vi "Unregister Object.vi"(6 "timeout (100 ms)":i32, 11 "Fully Qualified Name":string) -> (0 "timed out":bool)   [LabVIEW 2014, in "UniqueName.lvlib" / "UniqueName.lvclass"]
uses:
  UniqueName.lvclass
  Command.ctl
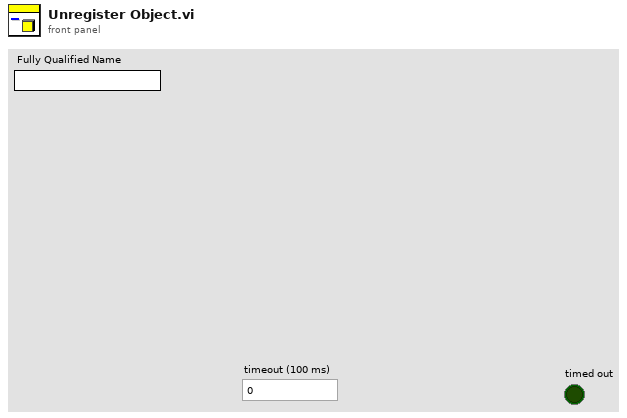
[diagram p1: front panel]
types:
  T1 = typedef "UniqueName.lvlib/UniqueName.lvclass/Command.ctl" = enum16{"Get", "Get All", "Set", "Delete", "Get Status", "Init", "Reserve Ownership", "Release Ownership", "Lock", "Unlock"}
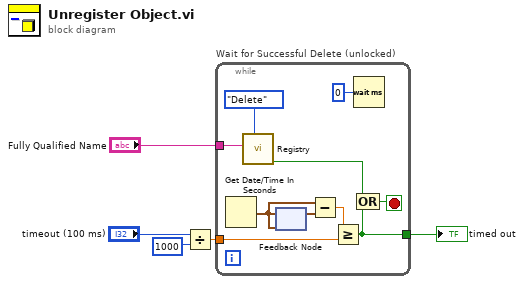
[diagram p0: block diagram]
diagram:
  n1 = Divide(x="timeout (100 ms)", y=1000) -> (x/y=w3:dbl)
  n2 = while "Wait for Successful Delete (unlocked)" {
    tunnel: w3 -> [w13]
    tunnel: [w7] -> w2
    tunnel: "Fully Qualified Name" -> [w6]
    stop <- w14 stop-if-true
    n3 = Get Date/Time In Seconds() -> (seconds since 1Jan1904=w11:timestamp)
    n4 = call "Registry.vi"("Command (Get)"=Command."Delete", "Search term (Get & Delete Operations)"=w6) -> ("Found or Completed?"=w8:bool)  [unwired: 5 in, 4 out]
    n5 = feedback-in #1(w11) -> ()
    n6 = feedback #1(w11) -> (w10:timestamp)
    n7 = Subtract(x=w11, y=w10) -> (x-y=w9:dbl)
    n8 = Greater Or Equal?(x=w9, y=w13) -> (x >= y?=w7:bool)
    n9 = Wait (ms)(milliseconds to wait=u32 0) -> ()  [unwired: 1 out]
    n10 = Compound Arithmetic op=OR(w8, w7) -> (w14:bool)
  }
  "timed out" <- w2
